vi "DiscArchiver.ProcConstructor.vi"(0 "i ref in":refnum<vi>, 3 "ms timeout (10000)":i32=10000, 5 "error in (no error)":errorcluster) -> (14 "i ref out":refnum<vi>, 17 "timed out":bool, 19 "error out":errorcluster)   [LabVIEW 2014, in "DiscArchiver.lvlib"]
doc: "This method allows to do initialization (to serve as a constructor for attributes). It is necessary, since the BaseProcess.i attribute is not initialized when the ClassName.constructor is executed."
uses:
  DiscArchiver.lvlib
  CSlibraries-extern/DimLVEvent/LVDimInterface/LVDimInterface.lvlib
  CS_Core/CSSystem/CSSystemLib/CSSystemLib.lvlib
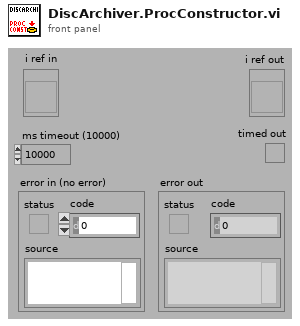
[diagram p1: front panel]
types:
  T1 = typedef "DiscArchiver.lvlib/DiscArchiver.i attribute.ctl" = cluster{"file prefix":string, "actual file":string, "nOfEvents":i32, "file":refnum<file>, "eventBuilder":string, "disc size alarm":bool, "dataDescription":string, "dataDescriptionURL":string, "eventDataURL":string, "headerID":dbl, "completeData":bool, "nOfEventsID":i32, "dataFileID":i32}
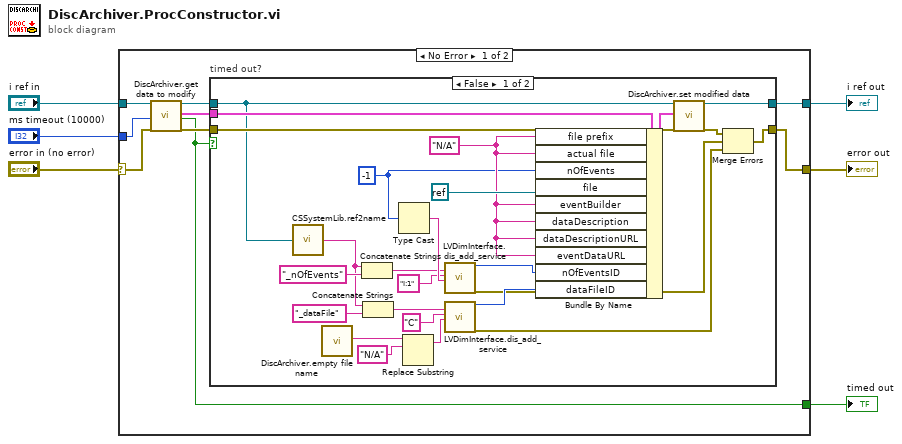
[diagram p0: block diagram]
diagram:
  n1 = case shown="No Error" "error in (no error)" {
    selector: "error in (no error)" -> [w7 w43]
    tunnel: "i ref in" -> [w15 w44]
    tunnel: [w14 w43] -> w5
    tunnel: [w13 w44] -> w4
    tunnel: "ms timeout (10000)" -> [w9 _]
    tunnel: [w8 _] -> w2
    frame No Error {
      n2 = call "DiscArchiver.get data to modify.vi"("i ref in"=w15, "ms timeout (10000)"=w9, "error in (no error)"=w7) -> ("i ref out"=w12:refnum<vi>, "i attribute"=w10:T1, "timed out"=w8:bool, "error out"=w11:errorcluster)  [unwired: 13 in]
      n3 = case "timed out?" shown="False" w8 {
        tunnel: [w21 w41] -> w14
        tunnel: [w40 w42] -> w13
        tunnel: w12 -> [w33 w42]
        tunnel: w11 -> [w39 w41]
        tunnel: w10 -> [w38 _]
        frame False {
          w32 = -1 ("# of items")
          w35 = "N/A" ("file body")
          n4 = call "CSSystemLib.ref2name.vi"("obj refnum"=w33) -> ("name"=w27:string)
          n5 = call "DiscArchiver.empty file name.vi"() -> ("emptyString"=w18:string)  [unwired: 19 in]
          n6 = Concatenate Strings(w27, "_nOfEvents" ("string")) -> (w28:string)
          n7 = Concatenate Strings(w27, "_dataFile" ("string")) -> (w25:string)
          n8 = Type Cast(x=w32) -> (*(type *) &x=w31:string)  [unwired: 1 in]
          n9 = Replace Substring(4:"N/A" ("substring (\"\")"), 5:w18) -> (1:w17:string)  [unwired: 2 in, 1 out]
          n10 = call "LVDimInterface.dis_add_service.vi"("serviceName"=w28, "typeDescriptor"="I:1", "data"=w31) -> ("my_serviceID"=w30:i32, "error out"=w20:errorcluster)  [unwired: 15 in]
          n11 = call "LVDimInterface.dis_add_service.vi"("serviceName"=w25, "typeDescriptor"="C", "data"=w17) -> ("my_serviceID"=w23:i32, "error out"=w19:errorcluster)  [unwired: 15 in]
          n12 = Bundle By Name(cluster=w38, "file prefix"=w35, "actual file"=w35, "nOfEvents"=w32, "file"=refnum<k0> refnum, "eventBuilder"=w35, "dataDescription"=w35, "dataDescriptionURL"=w35, "eventDataURL"=w35, "nOfEventsID"=w30, "dataFileID"=w23) -> (w37:T1)
          n13 = call "DiscArchiver.set modified data.vi"("i ref in"=w33, "i attribute"=w37, "error in (no error)"=w39) -> ("i ref out"=w40:refnum<vi>, "error out"=w22:errorcluster)  [unwired: 15 in]
          n14 = Merge Errors(w22, w20, w19) -> (w21:errorcluster)
        }
        frame True {
        }
      }
    }
    frame Error {
    }
  }
  "error out" <- w5
  "i ref out" <- w4
  "timed out" <- w2
